vi "Set plot legend.vi"(8 "error in (no error)":errorcluster, 9 "Data In":T3, 10 "Timeline":T1, 11 "XYGraph in":T2) -> (0 "error out":errorcluster, 3 "XYGraph out":T2)   [LabVIEW 2020, in "XGrapher.xctl"]
uses:
  XGrapher.xctl
  Data 1.ctl
  Typedefs/Xctrl-Data array.ctl
  Typedefs/Xcrtl-Data format definition.ctl
  Typedefs/Xctl-XY data type definition.ctl
  Typedefs/Xctrl-ROI type enum.ctl
  Typedefs/Xctrl-Waveform graph ref.ctl
  Typedefs/Xctrl-Timeline graph ref.ctl
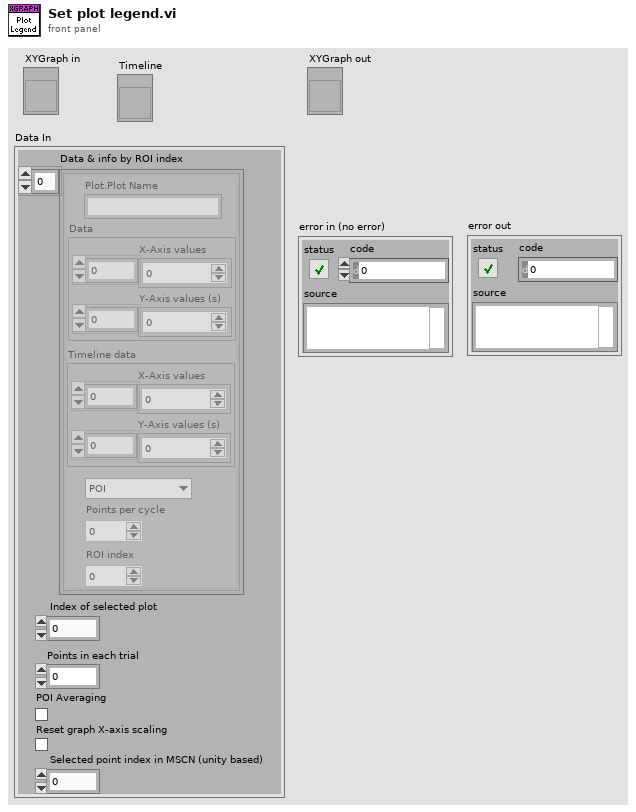
[diagram p1: front panel]
types:
  T1 = typedef "XGrapher.xctl/Xctrl-Timeline graph ref.ctl" = refnum<vi>
  T2 = typedef "XGrapher.xctl/Xctrl-Waveform graph ref.ctl" = refnum<vi>
  T3 = typedef "XGrapher.xctl/Data 1.ctl" = cluster{"Data & info by ROI index":T4, "Index of selected plot":u16, "Points in each trial":i32, "POI Averaging":bool, "Reset graph X-axis scaling":bool, "Selected point index in MSCN (unity based)":u16}
  T4 = typedef "Xctrl-Data array.ctl" = T5[]
  T5 = typedef "XGrapher.xctl/Xcrtl-Data format definition.ctl" = cluster{"Plot.Plot Name":string, "Data":T6, "Timeline data":T6, "Type":T7, "Points per cycle":u16, "ROI index":u16}
  T6 = typedef "XGrapher.xctl/Xctl-XY data type definition.ctl" = cluster{"X-Axis values":sgl[], "Y-Axis values (s)":sgl[]}
  T7 = typedef "Xctrl-ROI type enum.ctl" = enum16{"POI", "Mini-scan", "Group"}
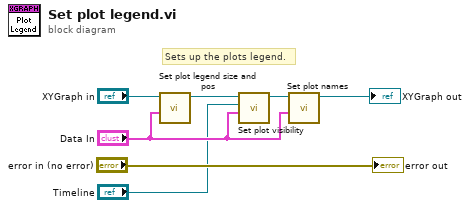
[diagram p0: block diagram]
diagram:
  # "Sets up the plots legend."
  n1 = call "Set plot legend size and pos.vi"("Data In (ordered by ROI index)"="Data In", "WaveformGraph in"="XYGraph in") -> ("WaveformGraph out"=w3:T2)  [unwired: 9 in]
  n2 = call "Set plot visibility.vi"("Data In"="Data In", "Timeline"="Timeline", "WaveformGraph in"=w3) -> ("WaveformGraph out"=w5:T2)  [unwired: 8 in]
  n3 = call "Set plot names.vi"("Data In (ordered by ROI index)"="Data In", "WaveformGraph in"=w5) -> ("WaveformGraph out"=→"XYGraph out":T2)  [unwired: 9 in]
  "error out" <- "error in (no error)"
